vi "LoadedCluster_toSetList_v5.vi"(0 "Devices queue":refnum<queue>, 1 "Layout Ref":refnum<vi>, 2 "Load w/o format? (F)":bool, 5 "Save Cluster":T1={"Version"="", "Devices"=[], "Select Layout"=0, "Layout:Strings And Values []"=[], "User defined functions"="-- -------------------------------------------------------------------------------------------\n-- The following functions are part of the \"standard load\" of functions and should not be messed with\n-- They are here for reference only.\n-- Please add any user functions above this comment\n-- -------------------------------------------------------------------------------------------\n\n-- Creates a linear ramp from A to B\nfunction LineRamp(f, Initial, Final)\n    return (1-f)*Initial + f*Final;\nend\n\n-- Creates an exponential ramp from A to B\nfunction ExpRamp(t, a, b, tau)\n   return (b - a*exp(tMax / tau) + (a-b)*exp(t/tau))/ ( 1 - exp(tMax / tau) );\nend\n\n-- Creates a sinewave\nfunction SinRamp(t,Offset,A,Freq, Phase)\n    return Offset + A * sin(2*pi*Freq*t + Phase)\nend\n\n-- Creates a blackman pulse\nfunction Blackman(f, Offset, A)\n    return Offset +  A*sqrt(0.5*cos(3.1415*(2*f-1))+0.08*cos(2*pi*(2*f-1))+0.42);\nend\n\n-- Creates a half-gauss ramp\nfunction HalfGaussRamp(t, a, b, Width)\n    local y;\n    y = exp(-(tMax^2)/Width^2);\n    y = (a -  b*y)/(1-y)  +  ((b-a)/(1-y))*exp(-((t-tMax)^2)/Width^2);\n    return y;\nend\n\n-- Creates an \"O'Hara\" ramp from A to B, for dipole evaporation\nfunction EvapRamp(t, a, b, tau)\n   local y;\n  y = log(a/b) / log(1+tMax/tau);\n  y = a * (1+t/tau)^(-y);\n  return y;\nend\n", "VariableManager"=refnum} {"Select Layout" items=["Default"]}, 7 "Table Ref in":refnum<vi>, 9 "VariableManagerRef":refnum<vi>, 11 "error in (no error)":errorcluster, 12 "Defer Updates? (T)":bool=TRUE, 13 "Reset Lua (T)":bool=TRUE) -> (3 "Loaded Version":string, 4 "Devices queue out":refnum<queue>, 6 "DevNums":i32[](array[numeric]), 8 "Col array":refnum<class "Column.lvclass">[](array[class]), 14 "User defined functions":string="-- -------------------------------------------------------------------------------------------\n-- The following functions are part of the \"standard load\" of functions and should not be messed with\n-- They are here for reference only.\n-- Please add any user functions above this comment\n-- -------------------------------------------------------------------------------------------\n\n-- Creates a linear ramp from A to B\nfunction LineRamp(f, Initial, Final)\n    return (1-f)*Initial + f*Final;\nend\n\n-- Creates an exponential ramp from A to B\nfunction ExpRamp(t, a, b, tau)\n   return (b - a*exp(tMax / tau) + (a-b)*exp(t/tau))/ ( 1 - exp(tMax / tau) );\nend\n\n-- Creates a sinewave\nfunction SinRamp(t,Offset,A,Freq, Phase)\n    return Offset + A * sin(2*pi*Freq*t + Phase)\nend\n\n-- Creates a blackman pulse\nfunction Blackman(f, Offset, A)\n    return Offset +  A*sqrt(0.5*cos(3.1415*(2*f-1))+0.08*cos(2*pi*(2*f-1))+0.42);\nend\n\n-- Creates a half-gauss ramp\nfunction HalfGaussRamp(t, a, b, Width)\n    local y;\n    y = exp(-(tMax^2)/Width^2);\n    y = (a -  b*y)/(1-y)  +  ((b-a)/(1-y))*exp(-((t-tMax)^2)/Width^2);\n    return y;\nend\n\n-- Creates an \"O'Hara\" ramp from A to B, for dipole evaporation\nfunction EvapRamp(t, a, b, tau)\n   local y;\n  y = log(a/b) / log(1+tMax/tau);\n  y = a * (1+t/tau)^(-y);\n  return y;\nend\n", 15 "error out":errorcluster)   [LabVIEW 2013]
doc: "Load devices and column array to SetList table from \"Save Cluster.\"\nAs is evident, this VI requires write access to Column array.\n\nOptionally, you may choose to \"Load w/o formatting.\" To use this option, you must first check that the new and existing device arrays are compatible with CompareDevices.vi."
uses:
  TypeDefs/SaveCluster.ctl
  VariableManagerCodes/VariableManager/VariableManager.lvclass
  DeviceVIs/Device/Device.lvclass
  <vilib>/Utility/miscctls.llb/LVStringsAndValuesArrayTypeDef_I32.ctl
  ColumnVIs/Column/Column.lvclass
  DeviceVIs/Pulseblaster/Pulseblaster.lvclass
  PackedLibraries/LuaEvaluatorAPI.lvlibp/API/t_Caching_Expression_Evaluator_Methods_Table.ctl
  VariableManagerCodes/API/VariableManagerAPI.lvlib
  PackedLibraries/LuaEvaluatorAPI.lvlibp
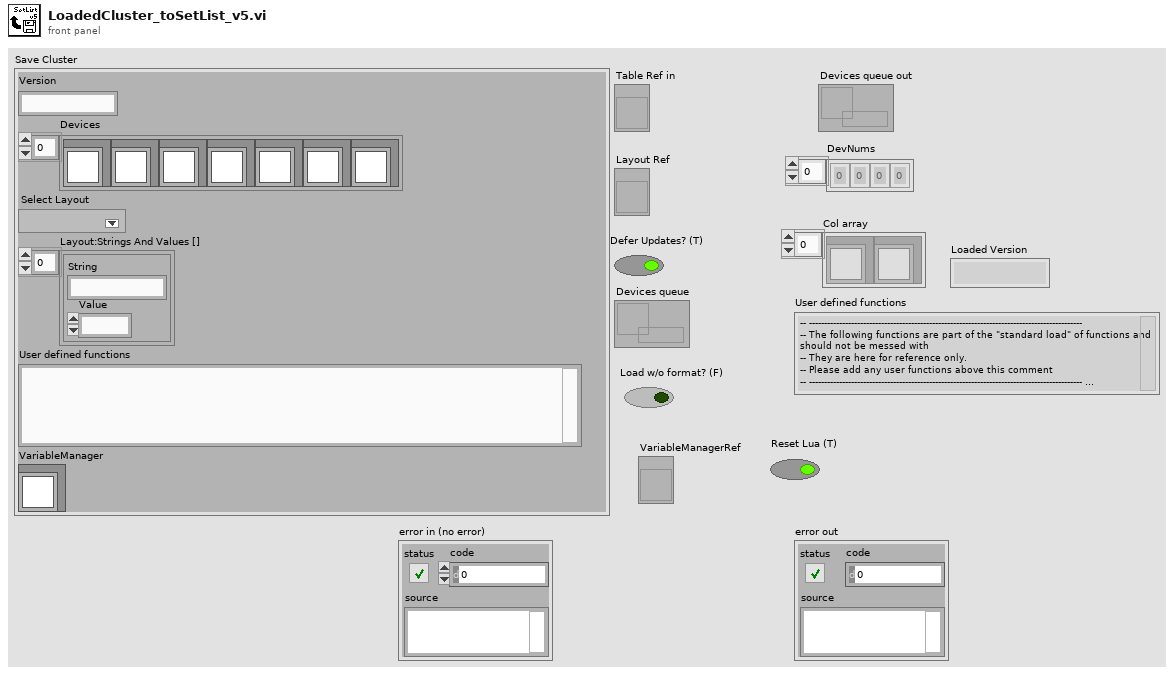
[diagram p1: front panel]
types:
  T1 = typedef "SaveCluster.ctl" = cluster{"Version":string, "Devices":refnum<class "Device.lvclass">[], "Select Layout":i32, "Layout:Strings And Values []":T2, "User defined functions":string, "VariableManager":refnum<class "VariableManager.lvclass">}
  T2 = typedef "LVStringsAndValuesArrayTypeDef_I32.ctl" = cluster{"String":string, "Value":i32}[]
  T3 = typedef "LuaEvaluatorAPI.lvlibp/t_Caching_Expression_Evaluator_Methods_Table.ctl" = enum16{"set", "get", "eval", "assign", "isvalid", "execute", "evaltable", "close"}
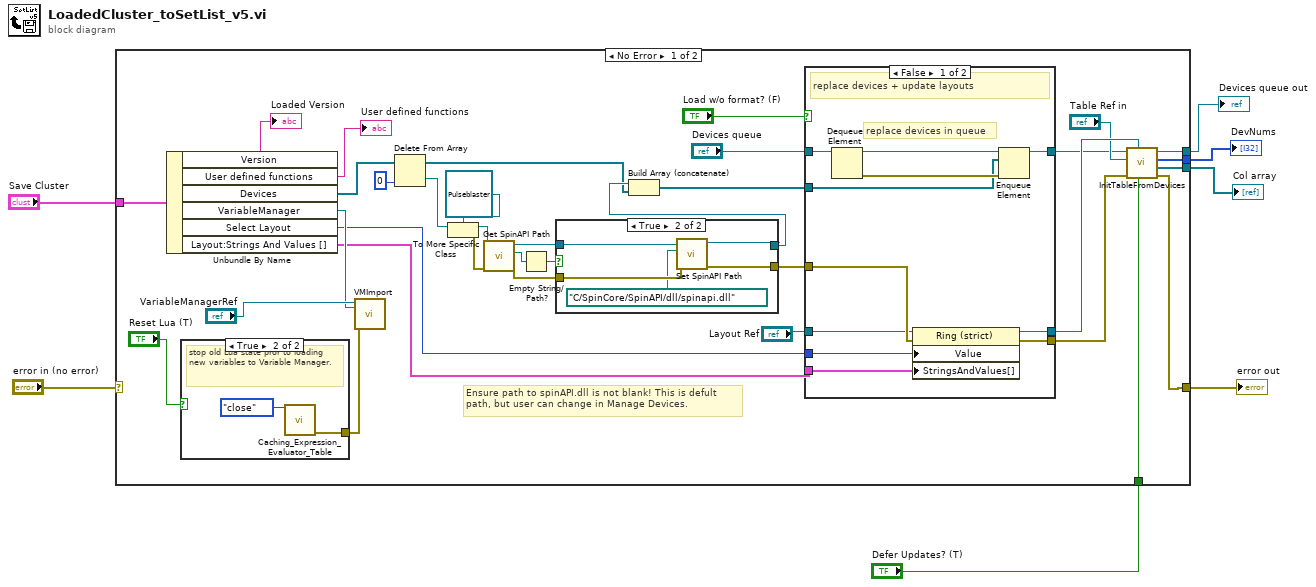
[diagram p0: block diagram]
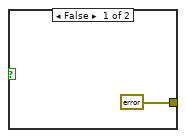
[diagram p2: hidden frame]
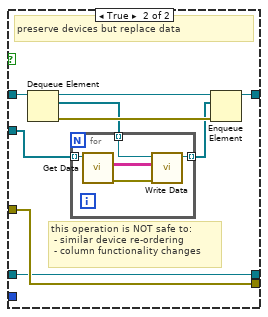
[diagram p3: hidden frame]
diagram:
  n1 = case shown="No Error" "error in (no error)" {
    selector: "error in (no error)" -> [_ w78]
    tunnel: "Save Cluster" -> [w42 _]
    tunnel: [w41 _] -> w1
    tunnel: [w40 _] -> w6
    tunnel: [w39 _] -> w5
    tunnel: [w38 w78] -> w4
    tunnel: "Defer Updates? (T)" -> [w37 _]
    frame No Error {
      # "Ensure path to spinAPI.dll is not blank! This is defult \npath, but user can change in Manage Devices."
      n2 = Unbundle By Name(w42) -> ("Version"=→"Loaded Version":string, "User defined functions"=→"User defined functions":string, "Devices"=w17:refnum<class "Device.lvclass">[], "VariableManager"=w32:refnum<class "VariableManager.lvclass">, "Select Layout"=w14:i32, "Layout:Strings And Values []"=w15:T2)
      n3 = case shown="True" "Reset Lua (T)" {
        tunnel: [errorcluster {"status"=FALSE, "code"=0, "source"=""} ("error out") w44] -> w30
        frame False {
        }
        frame True {
          # "stop old Lua state pror to loading\nnew variables to Variable Manager."
          n4 = call "Caching_Expression_Evaluator_Table.vi"("method"=t_Caching_Expression_Evaluator_Methods_Table."close") -> ("error out"=w44:errorcluster)  [unwired: 12 in, 2 out]
        }
      }
      n5 = call "VMImport.vi"("error in (no error)"=w30, "VariableManager"=w32, "VariableManagerRef in"="VariableManagerRef") -> ()  [unwired: 7 in, 2 out]
      n6 = Delete From Array(array=w17, index=0) -> (deleted portion=w25:refnum<class "Device.lvclass">, array with subset deleted=w16:refnum<class "Device.lvclass">[])  [unwired: 1 in]
      n7 = To More Specific Class(target class=refnum<class "Pulseblaster.lvclass"> refnum ("Pulseblaster.lvclass"), reference=w25) -> (specific class reference=w28:refnum<class "Pulseblaster.lvclass">, error out=w27:errorcluster)  [unwired: 1 in]
      n8 = call-dynamic "Get SpinAPI Path.vi"("error in (no error)"=w27, "Pulseblaster in"=w28) -> ("error out"=w20:errorcluster, "SpinAPI Path"=w23:path, "Pulseblaster out"=w21:refnum<class "Pulseblaster.lvclass">)  [unwired: 7 in]
      n9 = Empty String/Path?(string/path=w23) -> (empty?=w22:bool)
      n10 = case shown="True" w22 {
        tunnel: w21 -> [w71 w77]
        tunnel: w20 -> [w72 w76]
        tunnel: [w72 w75] -> w13
        tunnel: [w71 w74] -> w19
        frame False {
        }
        frame True {
          n11 = call-dynamic "Set SpinAPI Path.vi"("error in (no error)"=w76, "SpinAPI Path"=path "C:/SpinCore/SpinAPI/dll/spinapi.dll", "Pulseblaster in"=w77) -> ("error out"=w75:errorcluster, "Pulseblaster out"=w74:refnum<class "Pulseblaster.lvclass">)  [unwired: 7 in]
        }
      }
      n12 = Build Array (concatenate)(w19, w16) -> (w24:refnum<class "Device.lvclass">[])
      n13 = case shown="False" "Load w/o format? (F)" {
        tunnel: "Devices queue" -> [w56 w65]
        tunnel: [w55 w60] -> w35
        tunnel: [w52 w62] -> w31
        tunnel: w24 -> [w51 w59]
        tunnel: w15 -> [w50 _]
        tunnel: w14 -> [w49 _]
        tunnel: w13 -> [w48 w61]
        tunnel: [w47 w61] -> w12
        tunnel: "Layout Ref" -> [w46 w60]
        frame False {
          # "replace devices in queue"
          # "replace devices + update layouts"
          n14 = Dequeue Element(queue=w56) -> (queue out=w53:refnum<queue>, error out=w54:errorcluster)  [unwired: 2 in, 2 out]
          n15 = property on="Property Node" class="Ring (strict)"(reference=w46, error in=w48, "Value"=w49, "StringsAndValues[]"=w50) -> (reference out=w55:refnum<vi>, error out=w47:errorcluster)
          n16 = Enqueue Element(queue=w53, element=w51, error in (no error)=w54) -> (queue out=w52:refnum<queue>)  [unwired: 1 in, 2 out]
        }
        frame True {
          # "this operation is NOT safe to:\n - similar device re-ordering\n - column functionality changes"
          # "preserve devices but replace data"
          n17 = Dequeue Element(queue=w65) -> (queue out=w63:refnum<queue>, element=w58:refnum<class "Device.lvclass">[], error out=w64:errorcluster)  [unwired: 2 in, 1 out]
          n18 = for {
            tunnel: w59 -> [w68] mode=indexing
            tunnel: w58 -> [w67] mode=indexing
            tunnel: [w66] -> w57 mode=indexing
            n19 = call-dynamic "Get Data.vi"("Device in"=w68) -> ("error out"=w70:errorcluster, "Table Indicator"=w69:string[][])  [unwired: 7 in, 1 out]
            n20 = call-dynamic "Write Data.vi"("error in (no error)"=w70, "Data"=w69, "Device in"=w67) -> ("Device Out"=w66:refnum<class "Device.lvclass">)  [unwired: 7 in, 1 out]
          }
          n21 = Enqueue Element(queue=w63, element=w57, error in (no error)=w64) -> (queue out=w62:refnum<queue>)  [unwired: 1 in, 2 out]
        }
      }
      n22 = call "InitTableFromDevices.vi"("Defer Updates? (T)"=w37, "Layout Ref"=w35, "error in (no error)"=w12, "Table Ref in"="Table Ref in", "Devices queue"=w31) -> ("error out"=w38:errorcluster, "Col array"=w39:refnum<class "Column.lvclass">[], "DevNums"=w40:i32[], "Devices queue out"=w41:refnum<queue>)  [unwired: 3 in]
    }
    frame Error {
    }
  }
  "DevNums" <- w6
  "Col array" <- w5
  "error out" <- w4
  "Devices queue out" <- w1
